vi "host_logging_b2g1.vi"() -> ()   [LabVIEW 2011]
uses:
  <vilib>/addons/database/Connection.llb/Conn ObjectReference.ctl
  Output - Cluster b2g1.ctl
  <vilib>/Platform/TimedLoop/XDataNode/timing_clust.ctl
  <vilib>/Platform/TimedLoop/XDataNode/nitl_modes.ctl
  <vilib>/Platform/TimedLoop/XDataNode/wakeup.ctl
  <vilib>/Platform/TimedLoop/XDataNode/XDataNode.xnode
  <vilib>/Platform/TimedLoop/XDataNode/XDNodeRunTimeDep.lvlib
  <vilib>/addons/database/NI_Database_API.lvlib
panel:
  out "status":string
  in  "stop":bool caption="EXIT"
  out "Fehler":errorcluster
  in  "prefix for tables":string(combo)="B2G1"
  in  "interval [s]":u32=10 min=1 step=1
  in  "path":path
  # "B2G 1 DB Logging"
  # "database logging:"
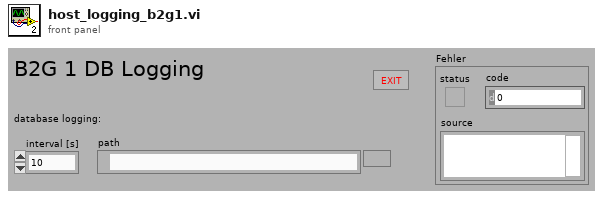
[diagram p1: front panel]
types:
  T1 = typedef "Output - Cluster b2g1.ctl" = cluster{"DFS-1 [dl]":u64, "FS-3 [l]":dbl, "DFS-1 [l/min]":dbl, "DS-1 [bar]":dbl, "V-10 ZU":bool, "V-14 ZU":bool, "FS-1 [l]":dbl, "FS-2 [l]":dbl, "TS-4 [°C]":dbl, "HS-1":bool, "V-13 [%]":u8, "V-15 [%]":u8, "P-4 [%]":u8, "P-5 [%]":u8, "Dosierung":bool, "MR Max Füllstand":bool, "MR Min Füllstand":bool, "Dosiermenge [l]":sgl, "V-14 AUF":bool, "V-10 AUF":bool, "T-1 Max Füllstand":bool, "T-1 Min Füllstand":bool, "T-2 Max Füllstand":bool, "T-2 Min Füllstand":bool, "pHS-1 [pH]":dbl, "P-4 RUN":bool, "P-5 RUN ":bool, "V-33 AUF":bool, "V-33 ZU":bool, "V-34 AUF":bool, "V-34 ZU":bool, "P-4 ERR":bool, "P-5 ERR":bool, "TS-5 [°C]":dbl, "TS-6 [°C]":dbl, "P-9 RUN":bool}
  T2 = typedef "NI_Database_API.lvlib/Conn ObjectReference.ctl" = refnum<k1>
  T3 = cluster{"file reference":refnum<file>, "file timing":i64, "db timing":i64, "DFS-1":u64, "db reference":T2, "P4 RUN":bool, "P5 RUN":bool, "file":bool, "db":bool, "data refnum":refnum<k21>, "input refnum":refnum<k21>, "feeding":bool, "feeding start volume":u64, "feeding start time":timestamp, "flashing":bool, "flashing start volume":u64, "flashing start time":timestamp, "V-33":bool, "V-34":bool, "V-15":u8, "V-13":u8, "P4 ERR":bool, "P5 ERR":bool, "V-14":bool, "V-10":bool, "prefix":string, "output cluster reading time":timestamp, "HS1":bool, "P9 RUN":bool}
  T4 = typedef "XDNodeRunTimeDep.lvlib/timing_clust.ctl" = cluster{"Expected End [f-1]":u64, "Actual End [f-1]":u64, "Finished Late? [f-1]":bool, "Expected End [i-1]":u64, "Actual End [i-1]":u64, "Finished Late? [i-1]":bool, "Expected Start [i]":u64, "Actual Start [i]":u64, "Expected Start [f]":u64, "Actual Start [f]":u64, "Source Name":string, "Structure Name":string, "Period":i64, "Deadline":i64, "Offset":i64, "Start":i64, "Priority":i32, "Timeout":i32, "Mode":T5, "Wakeup Reason":T6, "Error":errorcluster, "Source Type":string, "Secondary Source Type":string, "Global End Time":u64, "Global Start Time":u64, "Frame Duration":u64, "Iteration Duration":u64, "Assigned CPU":i32, "I/O Scan Engine Mode":u32}
  T5 = typedef "XDNodeRunTimeDep.lvlib/nitl_modes.ctl" = enum32{"No Change", "Process missed periods, maintain original phase", "Discard missed periods, maintain original phase", "Process missed periods, ignore original phase", "Discard missed periods, ignore original phase"}
  T6 = typedef "XDNodeRunTimeDep.lvlib/wakeup.ctl" = enum32{"Normal", "Aborted", "Asynchronous wakeup", "Timing source error", "Timed loop error", "Timeout"}
  T7 = enum32{"invalid app kind", "Development System", "Run Time System", "Student Edition", "Embedded LabVIEW", "Evaluation", "Custom"}
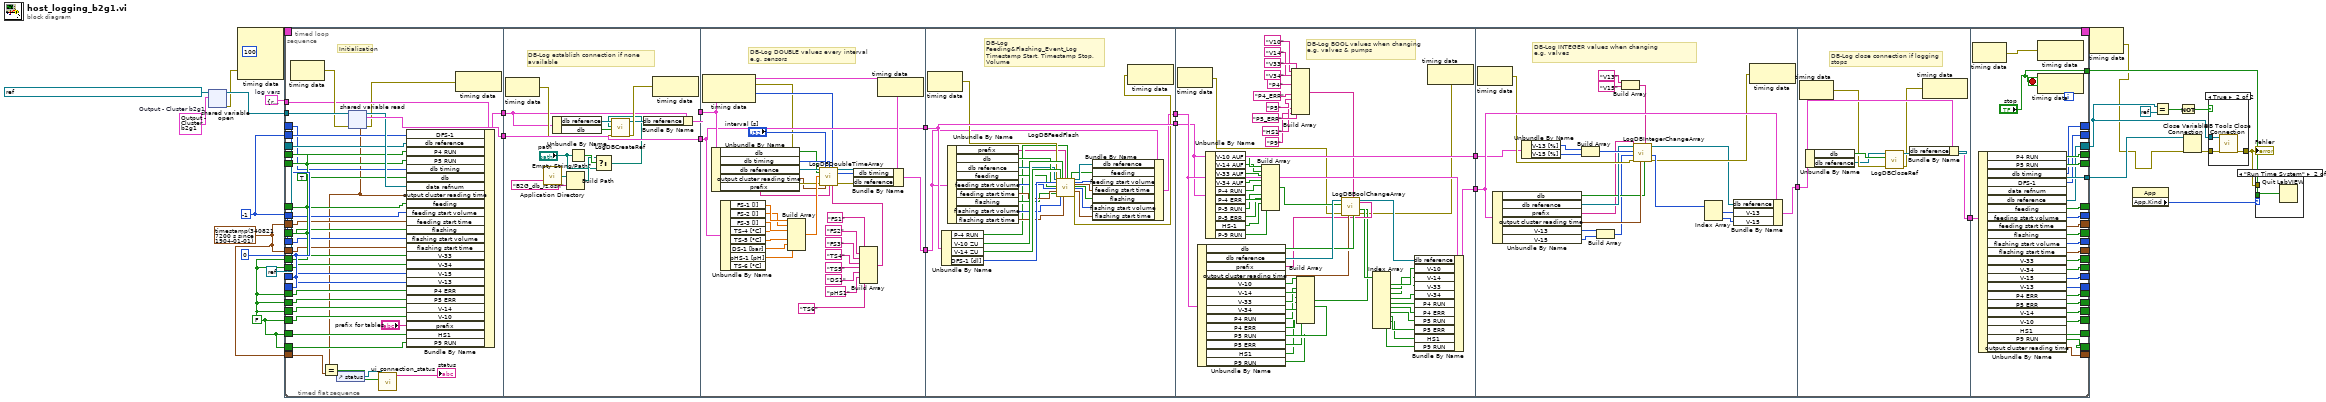
[diagram p0: block diagram]
diagram:
  w17 = T1 {"DFS-1 [dl]"=0, "FS-3 [l]"=0.0, "DFS-1 [l/min]"=0.0, "DS-1 [bar]"=0.0, "V-10 ZU"=FALSE, "V-14 ZU"=FALSE, "FS-1 [l]"=0.0, "FS-2 [l]"=0.0, "TS-4 [°C]"=0.0, "HS-1"=FALSE, "V-13 [%]"=0, "V-15 [%]"=0, "P-4 [%]"=0, "P-5 [%]"=0, "Dosierung"=FALSE, "MR Max Füllstand"=FALSE, "MR Min Füllstand"=FALSE, "Dosiermenge [l]"=0.0, "V-14 AUF"=FALSE, "V-10 AUF"=FALSE, "T-1 Max Füllstand"=FALSE, "T-1 Min Füllstand"=FALSE, "T-2 Max Füllstand"=FALSE, "T-2 Min Füllstand"=FALSE, "pHS-1 [pH]"=0.0, "P-4 RUN"=FALSE, "P-5 RUN "=FALSE, "V-33 AUF"=FALSE, "V-33 ZU"=FALSE, "V-34 AUF"=FALSE, "V-34 ZU"=FALSE, "P-4 ERR"=FALSE, "P-5 ERR"=FALSE, "TS-5 [°C]"=0.0, "TS-6 [°C]"=0.0, "P-9 RUN"=FALSE}  # Output - Cluster b2g1
  w20 = T3 {"file reference"=refnum, "file timing"=0, "db timing"=0, "DFS-1"=0, "db reference"=refnum, "P4 RUN"=FALSE, "P5 RUN"=FALSE, "file"=FALSE, "db"=FALSE, "data refnum"="ni.var.psp://10.27.40.21/variables - network - RT (separate)/data - network", "input refnum"="ni.var.psp://10.27.40.21/variables - network - RT (separate)/data - network", "feeding"=FALSE, "feeding start volume"=0, "feeding start time"=timestamp(0 s since 1904-01-01), "flashing"=FALSE, "flashing start volume"=0, "flashing start time"=timestamp(0 s since 1904-01-01), "V-33"=FALSE, "V-34"=FALSE, "V-15"=0, "V-13"=0, "P4 ERR"=FALSE, "P5 ERR"=FALSE, "V-14"=FALSE, "V-10"=FALSE, "prefix"="", "output cluster reading time"=timestamp(0 s since 1904-01-01), "HS1"=FALSE, "P9 RUN"=FALSE}  # log vars
  w2 = timestamp(3408217200 s since 1904-01-01) ("Time Stamp")
  w3 = FALSE ("P5")
  w15 = -1
  w14 = i64 0 ("Actual Start [i]")
  n1 = shared-variable-open(refnum<k21> "ni.var.psp://10.27.40.24/variables - b2g1/data - network - b2g1" ("output variable"), w17) -> (w18:refnum<k21>, w13:errorcluster)  [unwired: 2 in]
  n2 = node-c288(i64 100 ("Period"), w13) -> (w23:T4)  [unwired: 2 in]
  n3 = timed-loop {
    timing: w23 -> [_]
    timing-out: [_] -> w22
    shift-right: [w70] -> _
    shift-left: w14 -> [w71]
    tunnel: w20 -> [w69]
    shift-right: [w32] -> _
    shift-left: w15 -> [w61]
    shift-right: [w31] -> w6
    shift-left: refnum<k0> refnum -> [w68]
    shift-right: [w67] -> _
    shift-left: w3 -> [w66]
    shift-right: [w65] -> _
    shift-left: w3 -> [w64]
    tunnel: w18 -> [w63]
    tunnel: [w62] -> w5
    shift-right: [w60] -> _
    shift-left: w3 -> [w59]
    shift-right: [w58] -> _
    shift-left: w3 -> [w57]
    shift-right: [w56] -> _
    shift-left: w15 -> [w55]
    shift-right: [w54] -> _
    shift-left: w15 -> [w53]
    shift-right: [w52] -> _
    shift-left: w2 -> [w51]
    shift-right: [w50] -> _
    shift-left: w2 -> [w49]
    shift-right: [w48] -> _
    shift-left: w14 -> [w42]
    shift-right: [w47] -> _
    shift-left: w14 -> [w41]
    shift-right: [w46] -> _
    shift-left: w3 -> [w43]
    shift-right: [w45] -> _
    shift-left: w3 -> [w44]
    shift-right: [w40] -> _
    shift-left: w3 -> [w39]
    shift-right: [w38] -> _
    shift-left: w3 -> [w37]
    shift-right: [w36] -> _
    shift-left: w3 -> [w33]
    shift-right: [w35] -> _
    shift-left: w3 -> [w34]
    tunnel: [w30] -> w4
    shift-right: [w29] -> _
    shift-left: w3 -> [w28]
    shift-right: [w27] -> _
    shift-left: w3 -> [w26]
    shift-right: [w25] -> _
    shift-left: w2 -> [w24]
    stop <- "stop" stop-if-true
    n4 = timed-sequence {
      timing: _ -> [_]
      timing-out: _ -> [_]
      tunnel: w71 -> [w131]
      tunnel: [w130] -> w70
      tunnel: w69 -> [w129]
      tunnel: w68 -> [w128]
      tunnel: [w127] -> w67
      tunnel: w66 -> [w126]
      tunnel: [w125] -> w65
      tunnel: w64 -> [w124]
      tunnel: w63 -> [w119]
      tunnel: [w118] -> w62
      tunnel: w61 -> [w117]
      tunnel: [w114] -> w60
      tunnel: w59 -> [w113]
      tunnel: [w112] -> w58
      tunnel: w57 -> [w111]
      tunnel: [w110] -> w56
      tunnel: w55 -> [w109]
      tunnel: [w108] -> w54
      tunnel: w53 -> [w107]
      tunnel: [w106] -> w52
      tunnel: w51 -> [w105]
      tunnel: [w104] -> w50
      tunnel: w49 -> [w103]
      tunnel: [w100] -> w48
      tunnel: [w99] -> w47
      tunnel: [w98] -> w46
      tunnel: [w97] -> w45
      tunnel: w44 -> [w96]
      tunnel: w43 -> [w95]
      tunnel: w42 -> [w94]
      tunnel: w41 -> [w93]
      tunnel: [w90] -> w40
      tunnel: w39 -> [w89]
      tunnel: [w88] -> w38
      tunnel: w37 -> [w87]
      tunnel: [w86] -> w36
      tunnel: [w85] -> w35
      tunnel: w34 -> [w84]
      tunnel: w33 -> [w83]
      tunnel: [w80] -> w32
      tunnel: [w79] -> w31
      tunnel: [w78] -> w30
      tunnel: [w77] -> w29
      tunnel: w28 -> [w76]
      tunnel: [w75] -> w27
      tunnel: w26 -> [w74]
      tunnel: [w73] -> w25
      tunnel: w24 -> [w72]
      n5 = timed-flat-sequence {
        tunnel: w131 -> [w140]
        tunnel: [w164] -> w123
        tunnel: w129 -> [w148]
        tunnel: [w147] -> w121
        tunnel: w128 -> [w150]
        tunnel: w126 -> [w151]
        tunnel: w124 -> [w152]
        tunnel: w119 -> [w166]
        tunnel: w117 -> [w149]
        tunnel: w113 -> [w154]
        tunnel: w111 -> [w157]
        tunnel: w109 -> [w155]
        tunnel: w107 -> [w158]
        tunnel: w105 -> [w159]
        tunnel: w103 -> [w156]
        tunnel: w96 -> [w160]
        tunnel: w95 -> [w161]
        tunnel: w94 -> [w162]
        tunnel: w93 -> [w163]
        tunnel: w89 -> [w146]
        tunnel: w87 -> [w145]
        tunnel: w84 -> [w143]
        tunnel: w83 -> [w144]
        tunnel: w76 -> [w139]
        tunnel: w74 -> [w138]
        tunnel: w72 -> [w133]
        tunnel: w123 -> [w185]
        tunnel: [w185] -> w122
        tunnel: w121 -> [w181]
        tunnel: [w180] -> w120
        tunnel: w122 -> [w219]
        tunnel: [w219] -> w116
        tunnel: w120 -> [w220]
        tunnel: [w221] -> w115
        tunnel: w116 -> [w252]
        tunnel: [w252] -> w102
        tunnel: w115 -> [w240]
        tunnel: [w246] -> w101
        tunnel: w102 -> [w309]
        tunnel: w101 -> [w310]
        tunnel: [w311] -> w92
        tunnel: [w309] -> w81
        tunnel: w92 -> [w337]
        tunnel: [w338] -> w91
        tunnel: w81 -> [w318]
        tunnel: w91 -> [w349]
        tunnel: [w344] -> w82
        tunnel: [w362] -> w130
        tunnel: [w380] -> w127
        tunnel: [w379] -> w125
        tunnel: [w378] -> w118
        tunnel: [w377] -> w114
        tunnel: [w374] -> w112
        tunnel: [w376] -> w110
        tunnel: [w373] -> w108
        tunnel: [w372] -> w106
        tunnel: [w375] -> w104
        tunnel: [w369] -> w100
        tunnel: [w368] -> w99
        tunnel: [w370] -> w98
        tunnel: [w371] -> w97
        tunnel: [w367] -> w90
        tunnel: [w366] -> w88
        tunnel: [w365] -> w86
        tunnel: [w364] -> w85
        tunnel: w82 -> [w363]
        tunnel: [w361] -> w80
        tunnel: [w360] -> w79
        tunnel: ["stop"] -> w78
        tunnel: [w358] -> w77
        tunnel: [w357] -> w75
        tunnel: [w356] -> w73
        frame #0 {
          # "Initialisation"
          n6 = node-c288() -> (w165:errorcluster)  [unwired: 1 in]
          n7 = control-ref of="status"() -> (w135:refnum<vi>)
          n8 = shared-variable-read(w166, w165) -> (w153:refnum<k21>, w141:errorcluster, w164:T1, w132:timestamp)
          n9 = Equal?(x=w132, y=w133) -> (x = y?=w134:bool)
          n10 = call "ui_connection_status.vi"("Boolean"=w134, "String in"=w135) -> ("status"=→"status":string)  [unwired: 9 in]
          n11 = Bundle By Name(cluster=w148, "DFS-1"=w149, "db reference"=w150, "P4 RUN"=w151, "P5 RUN"=w152, "db timing"=w140, "db"=TRUE ("on/off"), "data refnum"=w153, "output cluster reading time"=w132, "feeding"=w154, "feeding start volume"=w155, "feeding start time"=w156, "flashing"=w157, "flashing start volume"=w158, "flashing start time"=w159, "V-33"=w160, "V-34"=w161, "V-15"=w162, "V-13"=w163, "P4 ERR"=w146, "P5 ERR"=w145, "V-14"=w144, "V-10"=w143, "prefix"="prefix for tables", "HS1"=w139, "P9 RUN"=w138) -> (w147:T3)
          n12 = node-c288(w141) -> ()  [unwired: 1 out]
        }
        frame #1 {
          # "DB-Log establish connection if none available"
          n13 = node-c288() -> (w183:errorcluster)  [unwired: 1 in]
          n14 = call <vilib>:"Application Directory.vi"() -> ("Application Directory"=w175:path)
          n15 = Unbundle By Name(w181) -> ("db reference"=w184:T2, "db"=w178:bool)
          n16 = Build Path(base path=w175, name or relative path="B2G_db_rz.dsn" ("Name of ini file 2")) -> (appended path=w176:path)
          n17 = Empty String/Path?(string/path="path") -> (empty?=w177:bool)
          n18 = Select(t=w176, s=w177, f="path") -> (s? t:f=w173:path)
          n19 = call "LogDBCreateRef.vi"("error in (no error)"=w183, "db"=w178, "Pfad in"=w173, "Refnum in"=w184) -> ("error out"=w182:errorcluster, "Refnum out"=w179:T2)  [unwired: 6 in]
          n20 = Bundle By Name(cluster=w181, "db reference"=w179) -> (w180:T3)
          n21 = node-c288(w182) -> ()  [unwired: 1 out]
        }
        frame #2 {
          # "DB-Log DOUBLE values every interval\ne.g. sensors"
          n22 = node-c288() -> (w194:errorcluster, w216:i64)  [unwired: 1 in]
          n23 = Unbundle By Name(w220) -> ("db"=w211:bool, "db timing"=w217:i64, "db reference"=w212:T2, "output cluster reading time"=w193:timestamp, "prefix"=w192:string)
          n24 = Unbundle By Name(w219) -> ("FS-1 [l]"=w202:dbl, "FS-2 [l]"=w201:dbl, "FS-3 [l]"=w200:dbl, "TS-4 [°C]"=w199:dbl, "TS-5 [°C]"=w198:dbl, "DS-1 [bar]"=w197:dbl, "pHS-1 [pH]"=w196:dbl)  [unwired: 1 out]
          n25 = Build Array(w202, w201, w200, w199, w198, w197, w196) -> (w195:dbl[])
          n26 = Build Array("FS1" ("table"), "FS2" ("table"), "FS3" ("table"), "TS4" ("table"), "TS5" ("table"), "DS1" ("table"), "pHS1" ("table"), "TS6" ("table")) -> (w203:string[])
          n27 = call "LogDBDoubleTimeArray.vi"("Refnum in"=w212, "db Interval [s]"="interval [s]", "db timing"=w217, "Actual Start [f] in"=w216, "db"=w211, "values"=w195, "error in (no error)"=w194, "Time Stamp"=w193, "prefix"=w192, "names"=w203) -> ("Refnum out"=w214:T2, "Actual Start [f] out"=w215:i64, "error out"=w213:errorcluster)  [unwired: 3 in]
          n28 = Bundle By Name(cluster=w220, "db timing"=w215, "db reference"=w214) -> (w221:T3)
          n29 = node-c288(w213) -> ()  [unwired: 1 out]
        }
        frame #3 {
          # "DB-Log\nFeeding&Flashing_Event_Log\nTimestamp Start, Timestamp Stop, Volume"
          n30 = node-c288() -> (w248:errorcluster)  [unwired: 1 in]
          n31 = Unbundle By Name(w252) -> ("P-4 RUN"=w229:bool, "V-10 ZU"=w250:bool, "V-14 ZU"=w249:bool, "DFS-1 [dl]"=w251:u64)
          n32 = Unbundle By Name(w240) -> ("prefix"=w228:string, "db"=w243:bool, "db reference"=w242:T2, "feeding"=w230:bool, "feeding start volume"=w241:u64, "feeding start time"=w239:timestamp, "flashing"=w231:bool, "flashing start volume"=w233:u64, "flashing start time"=w232:timestamp)
          n33 = call "LogDBFeedFlash.vi"("Refnum in"=w242, "value volume [dl]"=w251, "enable"=w243, "feeding"=w230, "feeding start volume"=w241, "feeding start time"=w239, "flashing"=w231, "error in"=w248, "valve t-2 close"=w249, "flashing start volume"=w233, "valve t-1 close"=w250, "flashing start time"=w232, "prefix"=w228, "Pump"=w229) -> ("feeding"=w244:bool, "Refnum out"=w245:T2, "feeding start volume"=w237:u64, "feeding start time"=w238:timestamp, "flashing"=w235:bool, "flashing start volume"=w234:u64, "flashing start time"=w236:timestamp, "error out"=w247:errorcluster)  [unwired: 6 in]
          n34 = Bundle By Name(cluster=w240, "db reference"=w245, "feeding"=w244, "feeding start volume"=w237, "feeding start time"=w238, "flashing"=w235, "flashing start volume"=w234, "flashing start time"=w236) -> (w246:T3)
          n35 = node-c288(w247) -> ()  [unwired: 1 out]
        }
        frame #4 {
          # "DB-Log BOOL values when changing\ne.g. valves & pumps"
          n36 = node-c288() -> (w267:errorcluster)  [unwired: 1 in]
          n37 = Unbundle By Name(w310) -> ("db"=w298:bool, "db reference"=w299:T2, "prefix"=w296:string, "output cluster reading time"=w297:timestamp, "V-10"=w285:bool, "V-14"=w284:bool, "V-33"=w283:bool, "V-34"=w282:bool, "P4 RUN"=w281:bool, "P4 ERR"=w280:bool, "P5 RUN"=w279:bool, "P5 ERR"=w278:bool, "HS1"=w265:bool, "P9 RUN"=w259:bool)
          n38 = Unbundle By Name(w309) -> ("V-10 AUF"=w276:bool, "V-14 AUF"=w275:bool, "V-33 AUF"=w274:bool, "V-34 AUF"=w273:bool, "P-4 RUN"=w272:bool, "P-4 ERR"=w271:bool, "P-5 RUN"=w270:bool, "P-5 ERR"=w269:bool, "HS-1"=w263:bool, "P-9 RUN"=w260:bool)
          n39 = Build Array(w276, w275, w274, w273, w272, w271, w270, w269, w263, w260) -> (w268:bool[])
          n40 = Build Array("V10" ("table"), "V14" ("table"), "V33" ("table"), "V34" ("table"), "P4" ("table"), "P4_ERR" ("table"), "P5" ("table"), "P5_ERR" ("table"), "HS1" ("table"), "P9" ("table")) -> (w300:string[])
          n41 = Build Array(w285, w284, w283, w282, w281, w280, w279, w278, w265, w259) -> (w277:bool[])
          n42 = call "LogDBBoolChangeArray.vi"("db"=w298, "names"=w300, "cluster reading time"=w297, "prefix"=w296, "error in (no error)"=w267, "shift reg in"=w277, "values"=w268, "db reference"=w299) -> ("error out"=w266:errorcluster, "shift reg out"=w294:bool[], "db reference out"=w295:T2)  [unwired: 1 in]
          n43 = Index Array(array=w294) -> (element #1=w293:bool, element #2=w292:bool, element #3=w291:bool, element #4=w290:bool, element #5=w289:bool, element #6=w288:bool, element #7=w287:bool, element #8=w286:bool, element #9=w264:bool, element #10=w258:bool)  [unwired: 10 in]
          n44 = Bundle By Name(cluster=w310, "db reference"=w295, "V-10"=w293, "V-14"=w292, "V-33"=w291, "V-34"=w290, "P4 RUN"=w289, "P4 ERR"=w288, "P5 RUN"=w287, "P5 ERR"=w286, "HS1"=w264, "P9 RUN"=w258) -> (w311:T3)
          n45 = node-c288(w266) -> ()  [unwired: 1 out]
        }
        frame #5 {
          # "DB-Log INTEGER values when changing\ne.g. valves"
          n46 = node-c288() -> (w327:errorcluster)  [unwired: 1 in]
          n47 = Unbundle By Name(w337) -> ("db"=w322:bool, "db reference"=w324:T2, "prefix"=w317:string, "output cluster reading time"=w325:timestamp, "V-13"=w321:u8, "V-15"=w320:u8)
          n48 = Unbundle By Name(w318) -> ("V-13 [%]"=w333:u8, "V-15 [%]"=w332:u8)
          n49 = Build Array(w333, w332) -> (w331:u8[])
          n50 = Build Array(w321, w320) -> (w319:u8[])
          n51 = Build Array("V13" ("table"), "V15" ("table")) -> (w334:string[])
          n52 = call "LogDBIntegerChangeArray.vi"("db"=w322, "names"=w334, "current time"=w325, "prefix"=w317, "error in (no error)"=w327, "shift reg in"=w319, "values"=w331, "Refnum in"=w324) -> ("error out"=w326:errorcluster, "shift reg out"=w328:u32[], "Refnum out"=w323:T2)  [unwired: 1 in]
          n53 = Index Array(array=w328) -> (element #1=w330:u32, element #2=w329:u32)  [unwired: 2 in]
          n54 = Bundle By Name(cluster=w337, "db reference"=w323, "V-13"=w330, "V-15"=w329) -> (w338:T3)
          n55 = node-c288(w326) -> ()  [unwired: 1 out]
        }
        frame #6 {
          # "DB-Log close connection if logging stops"
          n56 = node-c288() -> (w347:errorcluster)  [unwired: 1 in]
          n57 = Unbundle By Name(w349) -> ("db"=w348:bool, "db reference"=w345:T2)
          n58 = call "LogDBCloseRef.vi"("error in (no error)"=w347, "enable"=w348, "Refnum in"=w345) -> ("error out"=w346:errorcluster, "Refnum out"=w350:T2)  [unwired: 7 in]
          n59 = Bundle By Name(cluster=w349, "db reference"=w350) -> (w344:T3)
          n60 = node-c288(w346) -> ()  [unwired: 1 out]
        }
        frame #7 {
          n61 = node-c288() -> (w381:errorcluster)  [unwired: 1 in]
          n62 = Unbundle By Name(w363) -> ("P4 RUN"=w380:bool, "P5 RUN"=w379:bool, "db timing"=w362:i64, "DFS-1"=w361:u64, "data refnum"=w378:refnum<k21>, "db reference"=w360:T2, "feeding"=w377:bool, "feeding start volume"=w376:u64, "feeding start time"=w375:timestamp, "flashing"=w374:bool, "flashing start volume"=w373:u64, "flashing start time"=w372:timestamp, "V-33"=w371:bool, "V-34"=w370:bool, "V-15"=w369:u8, "V-13"=w368:u8, "P4 ERR"=w367:bool, "P5 ERR"=w366:bool, "V-14"=w365:bool, "V-10"=w364:bool, "HS1"=w358:bool, "P9 RUN"=w357:bool, "output cluster reading time"=w356:timestamp)
          n63 = node-c288(w381) -> ()  [unwired: 1 out]
        }
      }
    }
    n64 = node-c288() -> ()  [unwired: 1 in, 1 out]
    n65 = node-c288() -> ()  [unwired: 1 in, 1 out]
  }
  n66 = node-c288(w22) -> (w1:errorcluster)
  n67 = property class="App"() -> ("App.Kind"=w8:T7)  [unwired: 2 in, 2 out]
  n68 = Equal?(x=w6, y=refnum<k0> refnum) -> (x = y?=w12:bool)
  n69 = Not(x=w12) -> (.not. x?=w10:bool)
  n70 = Close Variable Connection(8:w1, 11:w5) -> (0:w9:errorcluster)
  n71 = case shown="True" w10 {
    tunnel: w9 -> [w389 w392]
    tunnel: w6 -> [_ w391]
    tunnel: [w389 w390] -> w7
    frame False {
    }
    frame True {
      n72 = call <vilib>:"DB Tools Close Connection.vi"("error in (no error)"=w392, "connection reference"=w391) -> ("error out"=w390:errorcluster)  [unwired: 5 in]
    }
  }
  "Fehler" <- w7
  n73 = case shown="\"Run Time System\"" w8 {
    tunnel: w7 -> [_ _ _]
    tunnel: w4 -> [_ w393 _]
    frame "invalid app kind", Default {
    }
    frame "Run Time System" {
      n74 = Quit LabVIEW(quit? (T)=w393) -> ()
    }
    frame "Development System" {
    }
  }
